vi "Traccia_Vin_Vout_2015.vi"() -> ()   [LabVIEW 2014]
doc: "Traccia_Vin_Vout\nUtilizza Vin_Vout e traccia una curva Vout vs Vin\n9/2011, 9/2015 vers. LV2014 \nFM & ADL"
uses:
  <vilib>/Utility/file.llb/Write To Spreadsheet File (DBL).vi
panel:
  in  "Fondo Scala AI0":dbl(ring)=10.0 items=["10"=10.0, "5"=5.0, "0.5"=0.5, "0.05"=0.05]
  in  "SALVA I DATI SU FILE":bool=TRUE caption="ON\nOFF"
  out "N. misura":i16
  out "Tensione di uscita in funzione della tensione di ingresso":cluster{dbl[], dbl[]}(graph)
  out "Vin (V)":dbl format="%_4g"
  out "Vout (V)":dbl format="%_4f"
  in  "Numero misure":i16=10 min=0 max=1000 step=1
  in  "Vmax(V)x":dbl=5.0 min=-10.0 max=10.0 step=0.1 format="%_4g"
  in  "Vmin(V)":dbl=-5.0 min=-10.0 max=10.0 step=0.1 format="%_4g"
  # "1) Scegliere il fondo scala dell'analog input: \n[10, 5, 0.5, 0.05]"
  # "Collegare il CB 22 (analog output) all'ingresso Vin  \ne il CB68 all'uscita Vout . \nLa terra del circuito (CB29) DEVE essere in comune alla terra della scheda."
  # "2) Selezionare il valore minimo e massimo della tensione di ingresso ed il numero di valori \n(equispaziati  tra gli estremi)"
  # "3) Premere la freccia bianca"
  # "Durante la misura gli indicatori  mostrano i valori di Vin e Vout ed il numero progressivo della misura"
  # "Sul grafico viene mostrata la tensione di uscita in funzione della tensione di ingresso."
  # "NO\nSI"
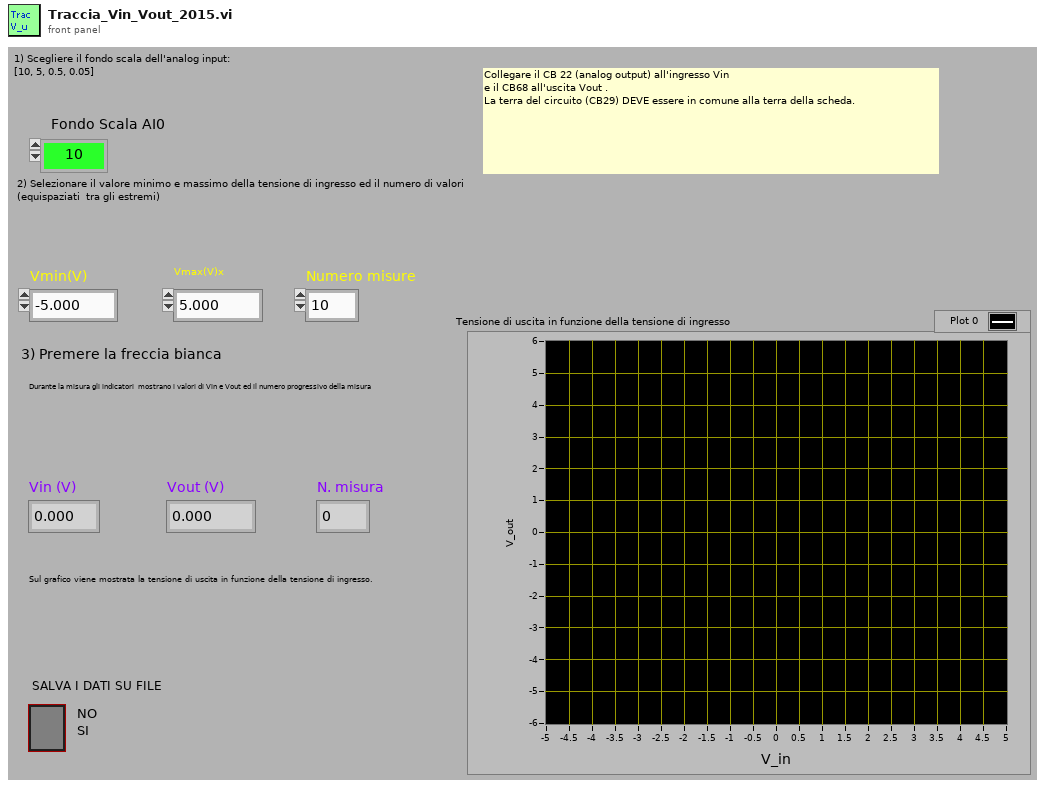
[diagram p1: front panel]
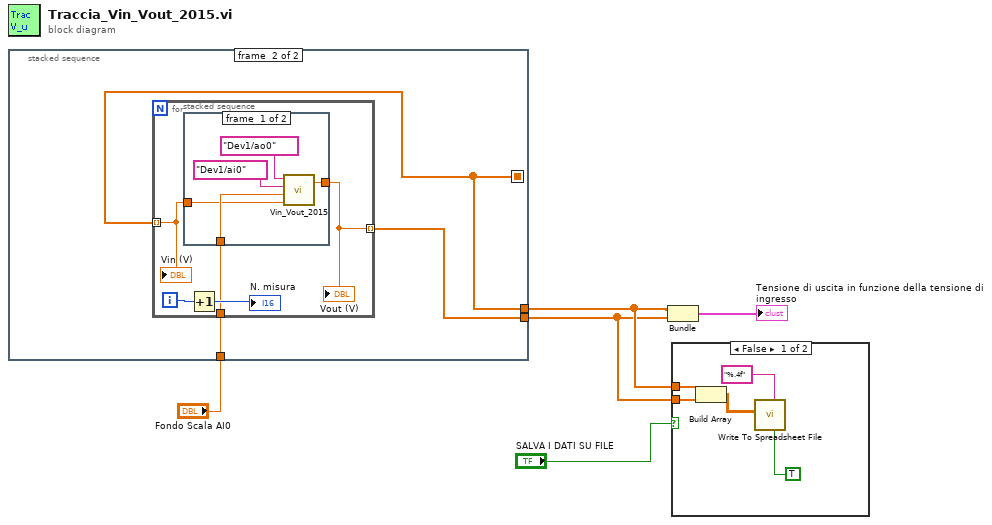
[diagram p0: block diagram]
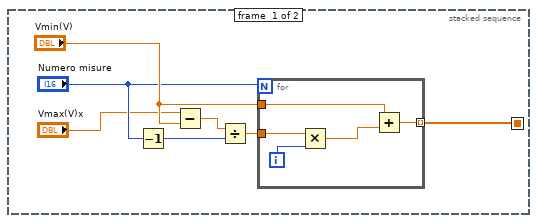
[diagram p3: hidden frame]
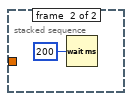
[diagram p4: hidden frame]
diagram:
  n1 = stacked-sequence {
    seq-local: [w8 _] -> [_ w18]
    tunnel: [_ w19] -> w3
    tunnel: [_ w18] -> w4
    tunnel: "Fondo Scala AI0" -> [_ w20]
    frame #0 {
      n2 = Decrement(x="Numero misure") -> (x-1=w11:i16)
      n3 = Subtract(x="Vmax(V)x", y="Vmin(V)") -> (x-y=w12:dbl)
      n4 = Divide(x=w12, y=w11) -> (x/y=w10:dbl)
      n5 = for {
        N: "Numero misure" -> [_]
        tunnel: "Vmin(V)" -> [w17]
        tunnel: [w16] -> w8 mode=indexing
        tunnel: w10 -> [w15]
        i -> [w14]
        n6 = Multiply(x=w15, y=w14) -> (x*y=w13:dbl)
        n7 = Add(x=w17, y=w13) -> (x+y=w16:dbl)
      }
    }
    frame #1 {
      n8 = for {
        tunnel: w18 -> [w25] mode=indexing
        tunnel: [w24] -> w19 mode=indexing
        tunnel: w20 -> [w21]
        i -> [w23]
        n9 = stacked-sequence {
          tunnel: w25 -> [w28 _]
          tunnel: [w30 _] -> w24
          tunnel: w21 -> [w29 _]
          frame #0 {
            n10 = call "Vin_Vout_2015.vi"("V in volt"=w28, "Fondo Scala 6024"=w29, "Canale Ingresso"=tag "Dev1/ai0", "Canale uscita"=tag "Dev1/ao0") -> ("mean Vout"=w30:dbl)  [unwired: 1 out]
          }
          frame #1 {
            n11 = Wait (ms)(milliseconds to wait=u32 200) -> ()  [unwired: 1 out]
          }
        }
        "Vout (V)" <- w24
        n12 = Increment(x=w23) -> (x+1=→"N. misura":i32)
        "Vin (V)" <- w25
      }
    }
  }
  n13 = Bundle(w4, w3) -> (→"Tensione di uscita in funzione della tensione di ingresso":cluster{dbl[], dbl[]})  [unwired: 1 in]
  n14 = case shown="False" "SALVA I DATI SU FILE" {
    tunnel: w3 -> [w36 _]
    tunnel: w4 -> [w35 _]
    frame False {
      n15 = Build Array(w35, w36) -> (w34:dbl[][])
      n16 = call-poly <vilib>:"Write To Spreadsheet File.vi"("transpose? (no:F)"=TRUE, "format (%.3f)"="%.4f", "2D data"=w34) -> ()  [unwired: 5 in, 1 out]
    }
    frame True {
    }
  }
